vi "ControlManual.vi"() -> ()   [LabVIEW 2020]
uses:
  VariablesGlobales.vi
panel:
  in  "Etiquetar":bool
  in  "Sellar":bool
  in  "Mezclar":bool
  in  "Encender Bomba 1":bool
  in  "Llenar Tanques":bool
  in  "Start":bool
  in  "Enceder Motor":bool
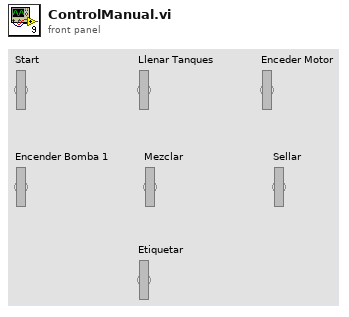
[diagram p1: front panel]
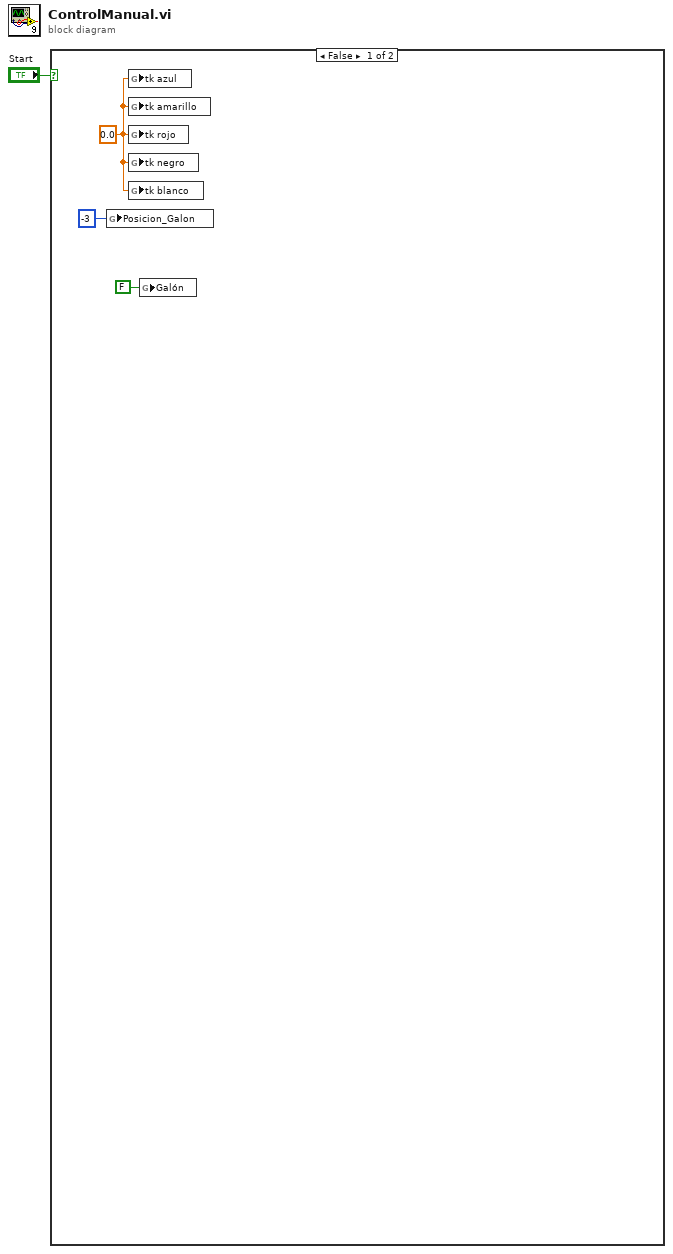
[diagram p0: block diagram]
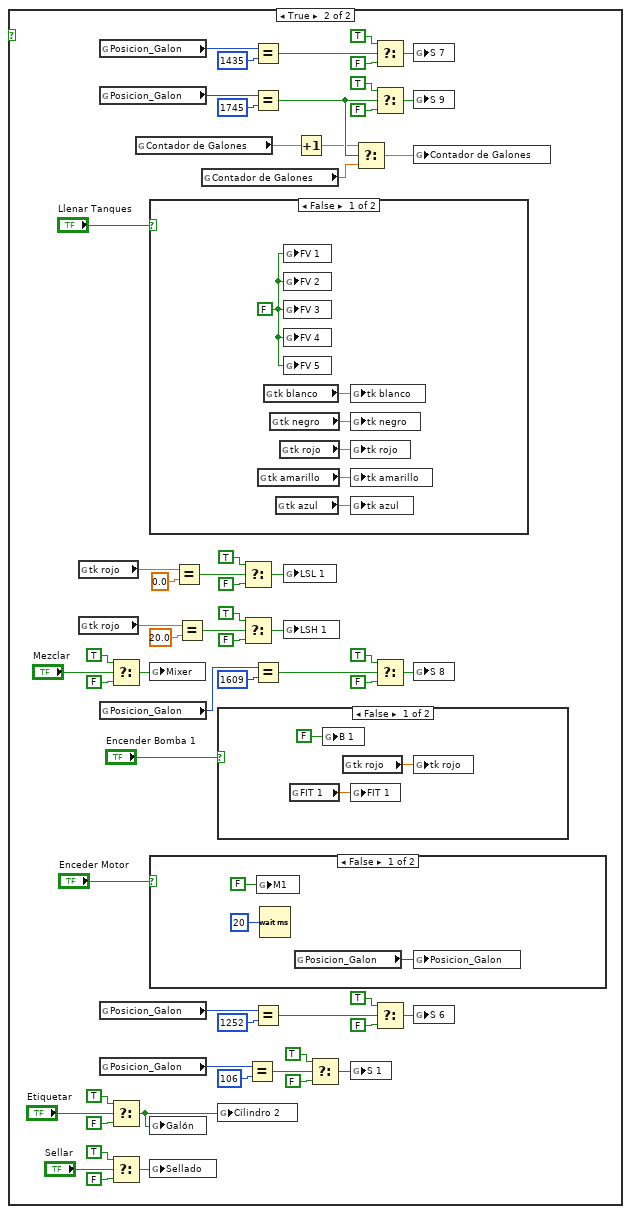
[diagram p2: hidden frame]
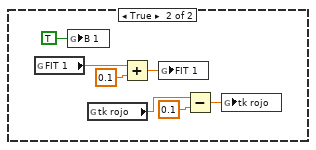
[diagram p3: hidden frame]
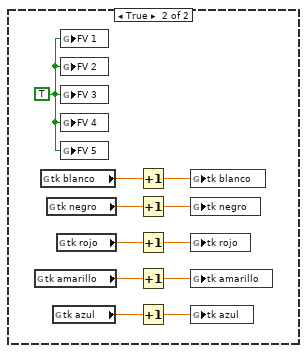
[diagram p4: hidden frame]
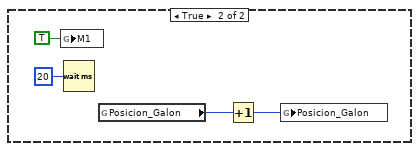
[diagram p5: hidden frame]
diagram:
  n1 = case shown="False" "Start" {
    frame False {
      w3 = 0.0 ("tk azul")
      n2 = global write "VariablesGlobales.vi" "Posicion_Galon"(-3 ("Posicion_Galon")) -> ()
      n3 = global write "VariablesGlobales.vi" "tk azul"(w3) -> ()
      n4 = global write "VariablesGlobales.vi" "tk amarillo"(w3) -> ()
      n5 = global write "VariablesGlobales.vi" "tk rojo"(w3) -> ()
      n6 = global write "VariablesGlobales.vi" "tk negro"(w3) -> ()
      n7 = global write "VariablesGlobales.vi" "tk blanco"(w3) -> ()
      n8 = global write "VariablesGlobales.vi" "Galón"(FALSE ("Galón")) -> ()
    }
    frame True {
      n9 = global read "VariablesGlobales.vi" "tk rojo"() -> (w63:dbl)
      n10 = global read "VariablesGlobales.vi" "tk rojo"() -> (w52:dbl)
      n11 = global read "VariablesGlobales.vi" "Posicion_Galon"() -> (w17:i32)
      n12 = global read "VariablesGlobales.vi" "Posicion_Galon"() -> (w16:i32)
      n13 = global read "VariablesGlobales.vi" "Posicion_Galon"() -> (w26:i32)
      n14 = global read "VariablesGlobales.vi" "Posicion_Galon"() -> (w39:i32)
      n15 = global read "VariablesGlobales.vi" "Posicion_Galon"() -> (w50:i32)
      n16 = Select(t=TRUE, s="Mezclar", f=FALSE) -> (s? t:f=w35:bool)
      n17 = Select(t=TRUE, s="Etiquetar", f=FALSE) -> (s? t:f=w28:bool)
      n18 = Select(t=TRUE, s="Sellar", f=FALSE) -> (s? t:f=w34:bool)
      n19 = global read "VariablesGlobales.vi" "Contador de Galones"() -> (w8:dbl)
      n20 = case shown="False" "Llenar Tanques" {
        frame False {
          w81 = FALSE ("FV 1")
          n21 = global read "VariablesGlobales.vi" "tk amarillo"() -> (w79:dbl)
          n22 = global read "VariablesGlobales.vi" "tk blanco"() -> (w76:dbl)
          n23 = global read "VariablesGlobales.vi" "tk negro"() -> (w77:dbl)
          n24 = global read "VariablesGlobales.vi" "tk azul"() -> (w80:dbl)
          n25 = global read "VariablesGlobales.vi" "tk rojo"() -> (w78:dbl)
          n26 = global write "VariablesGlobales.vi" "FV 1"(w81) -> ()
          n27 = global write "VariablesGlobales.vi" "FV 2"(w81) -> ()
          n28 = global write "VariablesGlobales.vi" "FV 3"(w81) -> ()
          n29 = global write "VariablesGlobales.vi" "FV 4"(w81) -> ()
          n30 = global write "VariablesGlobales.vi" "FV 5"(w81) -> ()
          n31 = global write "VariablesGlobales.vi" "tk blanco"(w76) -> ()
          n32 = global write "VariablesGlobales.vi" "tk negro"(w77) -> ()
          n33 = global write "VariablesGlobales.vi" "tk rojo"(w78) -> ()
          n34 = global write "VariablesGlobales.vi" "tk amarillo"(w79) -> ()
          n35 = global write "VariablesGlobales.vi" "tk azul"(w80) -> ()
        }
        frame True {
          w92 = TRUE ("FV 1")
          n36 = global read "VariablesGlobales.vi" "tk amarillo"() -> (w89:dbl)
          n37 = global read "VariablesGlobales.vi" "tk blanco"() -> (w82:dbl)
          n38 = global read "VariablesGlobales.vi" "tk negro"() -> (w85:dbl)
          n39 = global read "VariablesGlobales.vi" "tk azul"() -> (w90:dbl)
          n40 = global read "VariablesGlobales.vi" "tk rojo"() -> (w86:dbl)
          n41 = global write "VariablesGlobales.vi" "FV 1"(w92) -> ()
          n42 = global write "VariablesGlobales.vi" "FV 2"(w92) -> ()
          n43 = global write "VariablesGlobales.vi" "FV 3"(w92) -> ()
          n44 = global write "VariablesGlobales.vi" "FV 4"(w92) -> ()
          n45 = global write "VariablesGlobales.vi" "FV 5"(w92) -> ()
          n46 = Increment(x=w82) -> (x+1=w83:dbl)
          n47 = Increment(x=w85) -> (x+1=w84:dbl)
          n48 = Increment(x=w86) -> (x+1=w87:dbl)
          n49 = Increment(x=w89) -> (x+1=w88:dbl)
          n50 = Increment(x=w90) -> (x+1=w91:dbl)
          n51 = global write "VariablesGlobales.vi" "tk blanco"(w83) -> ()
          n52 = global write "VariablesGlobales.vi" "tk negro"(w84) -> ()
          n53 = global write "VariablesGlobales.vi" "tk rojo"(w87) -> ()
          n54 = global write "VariablesGlobales.vi" "tk amarillo"(w88) -> ()
          n55 = global write "VariablesGlobales.vi" "tk azul"(w91) -> ()
        }
      }
      n56 = global write "VariablesGlobales.vi" "Mixer"(w35) -> ()
      n57 = case shown="False" "Enceder Motor" {
        frame False {
          n58 = global write "VariablesGlobales.vi" "M1"(FALSE ("M1")) -> ()
          n59 = Wait (ms)(milliseconds to wait=u32 20) -> ()  [unwired: 1 out]
          n60 = global read "VariablesGlobales.vi" "Posicion_Galon"() -> (w94:i32)
          n61 = global write "VariablesGlobales.vi" "Posicion_Galon"(w94) -> ()
        }
        frame True {
          n62 = global write "VariablesGlobales.vi" "M1"(TRUE ("M1")) -> ()
          n63 = Wait (ms)(milliseconds to wait=u32 20) -> ()  [unwired: 1 out]
          n64 = global read "VariablesGlobales.vi" "Posicion_Galon"() -> (w98:i32)
          n65 = Increment(x=w98) -> (x+1=w97:i32)
          n66 = global write "VariablesGlobales.vi" "Posicion_Galon"(w97) -> ()
        }
      }
      n67 = global write "VariablesGlobales.vi" "Galón"(w28) -> ()
      n68 = global write "VariablesGlobales.vi" "Sellado"(w34) -> ()
      n69 = Equal?(x=w63, y=0.0) -> (x = y?=w61:bool)
      n70 = Equal?(x=w52, y=20.0) -> (x = y?=w54:bool)
      n71 = global read "VariablesGlobales.vi" "Contador de Galones"() -> (w9:dbl)
      n72 = case shown="False" "Encender Bomba 1" {
        frame False {
          n73 = global read "VariablesGlobales.vi" "FIT 1"() -> (w66:dbl)
          n74 = global write "VariablesGlobales.vi" "B 1"(FALSE ("B 1")) -> ()
          n75 = global read "VariablesGlobales.vi" "tk rojo"() -> (w67:dbl)
          n76 = global write "VariablesGlobales.vi" "FIT 1"(w66) -> ()
          n77 = global write "VariablesGlobales.vi" "tk rojo"(w67) -> ()
        }
        frame True {
          n78 = global read "VariablesGlobales.vi" "FIT 1"() -> (w70:dbl)
          n79 = global write "VariablesGlobales.vi" "B 1"(TRUE ("B 1")) -> ()
          n80 = global read "VariablesGlobales.vi" "tk rojo"() -> (w73:dbl)
          n81 = Add(x=w70, y=0.1) -> (x+y=w69:dbl)
          n82 = global write "VariablesGlobales.vi" "FIT 1"(w69) -> ()
          n83 = Subtract(x=w73, y=0.1) -> (x-y=w74:dbl)
          n84 = global write "VariablesGlobales.vi" "tk rojo"(w74) -> ()
        }
      }
      n85 = global write "VariablesGlobales.vi" "Cilindro 2"(w28) -> ()
      n86 = Select(t=TRUE, s=w61, f=FALSE) -> (s? t:f=w58:bool)
      n87 = Select(t=TRUE, s=w54, f=FALSE) -> (s? t:f=w57:bool)
      n88 = Equal?(x=w50, y=106) -> (x = y?=w47:bool)
      n89 = Equal?(x=w17, y=1435) -> (x = y?=w20:bool)
      n90 = Equal?(x=w16, y=1745) -> (x = y?=w11:bool)
      n91 = Equal?(x=w26, y=1609) -> (x = y?=w23:bool)
      n92 = Equal?(x=w39, y=1252) -> (x = y?=w42:bool)
      n93 = global write "VariablesGlobales.vi" "LSL 1"(w58) -> ()
      n94 = global write "VariablesGlobales.vi" "LSH 1"(w57) -> ()
      n95 = Increment(x=w8) -> (x+1=w7:dbl)
      n96 = Select(t=TRUE, s=w47, f=FALSE) -> (s? t:f=w45:bool)
      n97 = global write "VariablesGlobales.vi" "S 1"(w45) -> ()
      n98 = Select(t=w7, s=w11, f=w9) -> (s? t:f=w10:dbl)
      n99 = Select(t=TRUE, s=w20, f=FALSE) -> (s? t:f=w21:bool)
      n100 = Select(t=TRUE, s=w11, f=FALSE) -> (s? t:f=w13:bool)
      n101 = Select(t=TRUE, s=w23, f=FALSE) -> (s? t:f=w22:bool)
      n102 = Select(t=TRUE, s=w42, f=FALSE) -> (s? t:f=w44:bool)
      n103 = global write "VariablesGlobales.vi" "S 7"(w21) -> ()
      n104 = global write "VariablesGlobales.vi" "S 9"(w13) -> ()
      n105 = global write "VariablesGlobales.vi" "Contador de Galones"(w10) -> ()
      n106 = global write "VariablesGlobales.vi" "S 8"(w22) -> ()
      n107 = global write "VariablesGlobales.vi" "S 6"(w44) -> ()
    }
  }
